vi "Ping_test.vi"   [LabVIEW 2018]
types:
  T1 = cluster{"function type":enum16{"none", "init", "write", "read"}, "Desc str":string, "function name":string, "error constant":errorcluster}
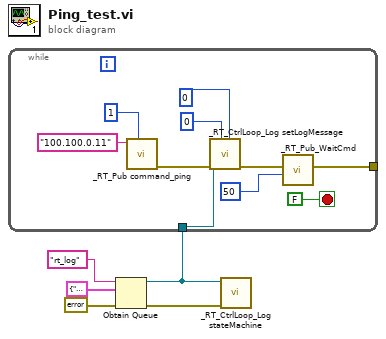
[diagram p0: block diagram]
diagram:
  n1 = Obtain Queue(name (unnamed)="rt_log", element data type=T1 {"function type"=enum."none", "Desc str"="", "function name"="", "error constant"={"status"=FALSE, "code"=0, "source"=""}}, error in (no error)=errorcluster {"status"=FALSE, "code"=0, "source"=""} ("Error in")) -> (queue out=w1:refnum<queue>, error out=w3:errorcluster)  [unwired: 2 in, 1 out]
  n2 = while {
    tunnel: [w9] -> _
    tunnel: w1 -> [w6]
    stop <- FALSE stop-if-true
    n3 = call "_RT_Pub command_ping.vi"("Loop Times"=1, "PCIP String"="100.100.0.11") -> ("error out"=w12:errorcluster)  [unwired: 9 in]
    n4 = call "_RT_CtrlLoop_Log setLogMessage.vi"(5:u16 0 ("N2"), "system type"=u16 0 ("N1"), "error in"=w12, "RTLogQueue in"=w6) -> ("error out"=w10:errorcluster)  [unwired: 6 in, 1 out]
    n5 = call "_RT_Pub_WaitCmd.vi"("milliseconds to wait"=u32 50, "error in (no error)"=w10) -> ("error out"=w9:errorcluster)  [unwired: 9 in]
  }
  n6 = call "_RT_CtrlLoop_Log stateMachine.vi"("error in (no error)"=w3, "RTLogQueue in"=w1) -> ()  [unwired: 9 in, 1 out]
